vi "2-EvenOdd.vi"() -> ()   [LabVIEW 2014]
panel:
  out "iteration":dbl
  out "Even":bool
  out "Odd":bool
  in  "stop":bool
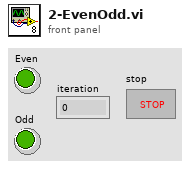
[diagram p1: front panel]
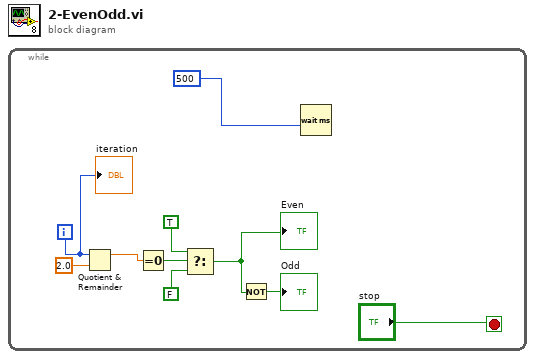
[diagram p0: block diagram]
diagram:
  n1 = while {
    i -> [w1]
    stop <- "stop" stop-if-true
    n2 = Quotient & Remainder(x=w1, y=2.0) -> (x-y*floor(x/y)=w7:dbl)  [unwired: 1 out]
    n3 = Equal To 0?(x=w7) -> (x = 0?=w8:bool)
    n4 = Select(t=TRUE, s=w8, f=FALSE) -> (s? t:f=w3:bool)
    "Even" <- w3
    n5 = Not(x=w3) -> (.not. x?=→"Odd":bool)
    n6 = Wait (ms)(milliseconds to wait=500) -> ()  [unwired: 1 out]
    "iteration" <- w1
  }
